vi "ANN_GetPosture.vi"(9 "quaternion":sgl[](array[numeric]), 11 "position":sgl[](array[numeric])) -> (3 "vehicle status":T1)   [LabVIEW 2017]
doc: "This VI returns the current posture information (x, y, O) of the DaNI robot from the simulator. In real world applications, you can acquire posture information from sensors."
uses:
  VehiclePosture.ctl
  <vilib>/Analysis/_algsub.llb/Vector Norm.vi
  <vilib>/Analysis/_algsub.llb/Real Vector Norm.vi
  <vilib>/robotics/Simulator/NI_Robotics_Simulator.lvlib
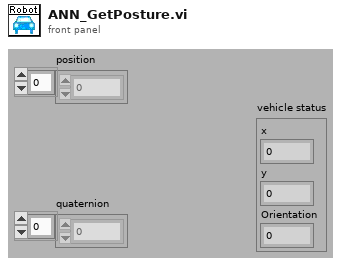
[diagram p1: front panel]
types:
  T1 = typedef "VehiclePosture.ctl" = cluster{"x":dbl, "y":dbl, "Orientation":dbl}
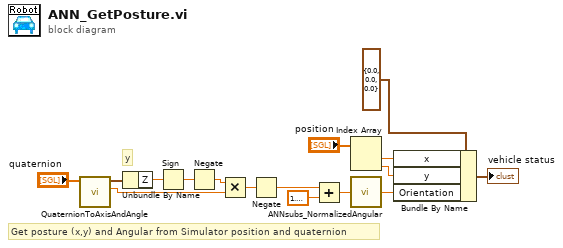
[diagram p0: block diagram]
diagram:
  # "Get posture (x,y) and Angular from Simulator position and quaternion"
  # "y"
  n1 = call <vilib>:"QuaternionToAxisAndAngle.vi"("Quaternion"="quaternion") -> ("Angle"=w1:dbl, "Axis"=w2:cluster{"X":dbl, "Y":dbl, "Z":dbl})  [unwired: 8 in, 1 out]
  n2 = Unbundle By Name(w2) -> ("Z"=w14:dbl)
  n3 = Sign(1:w14) -> (0:w13:dbl)
  n4 = Negate(x=w13) -> (-x=w12:dbl)
  n5 = Multiply(x=w12, y=w1) -> (x*y=w9:dbl)
  n6 = Negate(x=w9) -> (-x=w7:dbl)
  n7 = Add(x=w7, y=1.5707963267948966) -> (x+y=w6:dbl)
  n8 = Index Array(array="position") -> (element #1=w5:sgl, element #2=w4:sgl)  [unwired: 2 in]
  n9 = call "ANNsubs_NormalizedAngular.vi"("Delta angle"=w6) -> ("Delta angle out"=w11:dbl)
  n10 = Bundle By Name(cluster=T1 {"x"=0.0, "y"=0.0, "Orientation"=0.0} ("VehiclePosture"), "x"=w5, "y"=w4, "Orientation"=w11) -> (→"vehicle status":T1)
